vi "rms_voltage_to_current.vi"(11 "RMS [V]":dbl[](array[numeric])) -> (3 "RMS[A]":dbl[](array[numeric]))   [LabVIEW 2025, in "LabJackEKG.lvlib"]
uses:
  LabJackEKG.lvlib
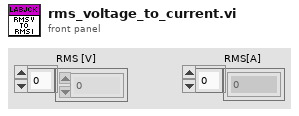
[diagram p1: front panel]
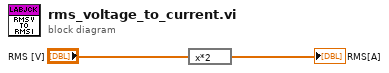
[diagram p0: block diagram]
diagram:
  n1 = expression code="x*2"("RMS [V]") -> (→"RMS[A]":dbl[])
